vi "SaveCorner (SubVI).vi"(0 "Module record filename":path, 1 "Temperature":dbl, 2 "Write to file":bool, 5 "Data strings":T1, 7 "Module corner image filename":path, 9 "Image of corner":T2, 11 "error in (no error)":errorcluster) -> (15 "error out":errorcluster)   [LabVIEW 2016]
uses:
  <vilib>/vision/Image Controls.llb/IMAQ Image.ctl
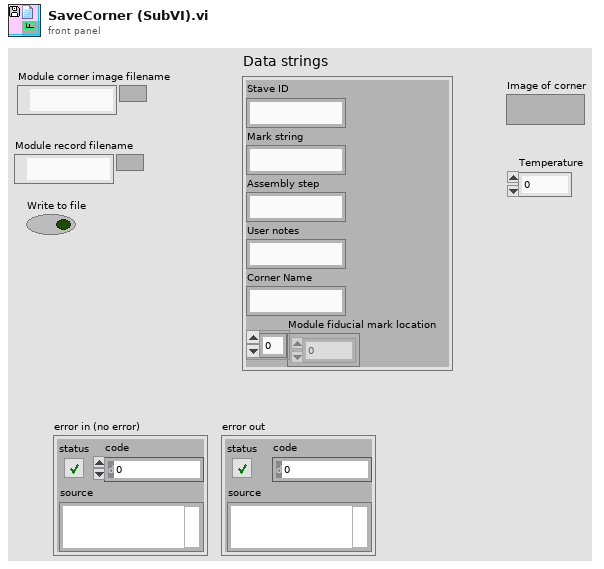
[diagram p1: front panel]
types:
  T1 = cluster{"Stave ID":string, "Mark string":string, "Assembly step":string, "User notes":string, "Corner Name":string, "Module fiducial mark location":dbl[]}
  T2 = typedef "IMAQ Image.ctl" = refnum<image>
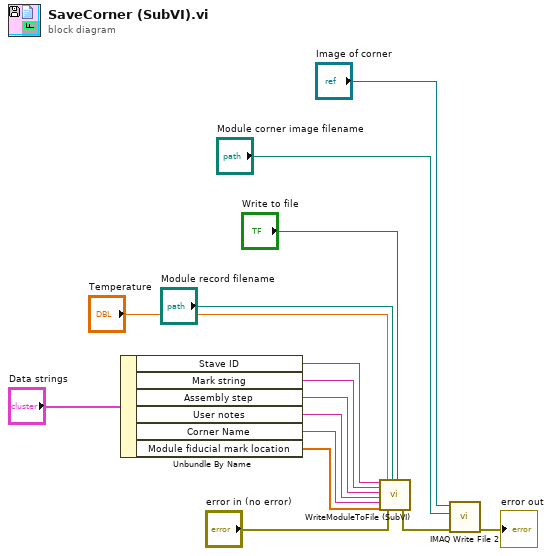
[diagram p0: block diagram]
diagram:
  n1 = Unbundle By Name("Data strings") -> ("Stave ID"=w7:string, "Mark string"=w6:string, "Assembly step"=w5:string, "User notes"=w3:string, "Corner Name"=w2:string, "Module fiducial mark location"=w4:dbl[])
  n2 = call "WriteModuleToFile (SubVI).vi"("Stave ID"=w7, "Mark used for tracking"=w6, "Assembly step"=w5, "User notes"=w3, "Current corner"=w2, "Fiducial Mark Position"=w4, "Temperature"="Temperature", "error in (no error)"="error in (no error)", "Module reports file path"="Module record filename", "Write to file"="Write to file") -> ("error out"=w14:errorcluster)  [unwired: 9 in]
  n3 = call-poly "IMAQ Write File 2"("error in (no error)"=w14, "File Path"="Module corner image filename", "Image"="Image of corner") -> ("error out"=→"error out":errorcluster)  [unwired: 7 in, 1 out]
